vi "log analysis_gps.vi"() -> ()   [LabVIEW 2019] (continued)
11.7738,22.3000,0.0889,-0.2912,-0.0157,0.137018151,-1.334468427,280.534881050,0.4569,0.2986,0.5535,0.1156,0.0931,0.0772,0.0995,0.1050,4.8407,0f000001,0*4cc88e7a\n\tsystem status\tnormal 2 27.900000 0 0\trobot status\t339.401194\t32.171850\t11.773800\t0.137018\t-1.334468\t169.465119\t0.367000\t-0.094000\n\t\n15:29:25.3\tlog_raw\tgps_raw\t\tsystem status\tnormal 2 27.900000 0 0\trobot status\t339.281067\t32.209175\t11.771900\t0.263752\t-1.166349\t169.684950\t0.262000\t0.068000\n\t\n15:29:25.8\tlog_raw\tgps_raw\t#DUALANTENNAHEADINGA,USB3,0,50.0,FINESTEERING,2107,282583.800,02000000,d426,15824;SOL_COMPUTED,L1_FLOAT,-1.000000000,298.425811768,-39.243469238,0.0,360.000000000,180.000000000,\"631T\",12,4,4,4,04,00,20,00*99234be7\n\tsystem status\tnormal 2 27.900000 0 0\trobot status\t339.146863\t32.249468\t11.770100\t0.297724\t-0.965095\t169.902613\t0.288000\t0.022000\n\t\n15:29:26.3\tlog_raw\tgps_raw\t#INSPVAXA,USB3,0,50.0,FINESTEERING,2107,282584.350,02000000,471d,15824;INS_ALIGNMENT_COMPLETE,INS_RTKFIXED,37.37042121578,126.72466218098,11.7682,22.3000,0.0908,-0.2905,-0.0097,0.228953863,-0.969786949,279.904204523,0.4542,0.2977,0.5520,0.1156,0.0930,0.0771,0.0995,0.1050,4.8423,0f000001,0*25d05607\n\tsystem status\tnormal 2 27.900000 0 0\trobot status\t339.009591\t32.288365\t11.768300\t0.251734\t-1.037795\t170.066210\t0.264000\t0.046000\n\t\n15:29:26.8\tlog_raw\tgps_raw\t#DUALANTENNAHEADINGA,USB3,0,50.0,FINESTEERING,2107,282584.800,02000000,d426,15824;SOL_COMPUTED,L1_FLOAT,-1.000000000,317.813751221,-55.080688477,0.0,360.000000000,180.000000000,\"631T\",14,4,4,4,04,00,20,00*482add9e\n\tsystem status\tnormal 2 27.900000 0 0\trobot status\t338.871429\t32.326322\t11.766900\t0.026488\t-1.197862\t170.161249\t0.289000\t0.009000\n\t\n15:29:27.3\tlog_raw\tgps_raw\t#DUALANTENNAHEADINGA,USB3,0,47.5,FINESTEERING,2107,282585.300,02008000,d426,15824;SOL_COMPUTED,L1_FLOAT,-1.000000000,279.031005859,-12.437835693,0.0,360.000000000,180.000000000,\"631T\",14,4,4,4,04,00,20,00*e33ff00b\n\tsystem status\tnormal 2 28.000000 0 0\trobot status\t338.733347\t32.363284\t11.765300\t-0.055749\t-1.396296\t170.255636\t0.233000\t0.094000\n\t\n15:29:27.8\tlog_raw\tgps_raw\t#DUALANTENNAHEADINGA,USB3,0,47.5,FINESTEERING,2107,282585.800,02008000,d426,15824;SOL_COMPUTED,L1_FLOAT,-1.000000000,288.534484863,-28.210021973,0.0,360.000000000,180.000000000,\"631T\",14,4,4,4,04,00,20,00*75d90e5f\n\tsystem status\tnormal 2 28.000000 0 0\trobot status\t338.595043\t32.400275\t11.762200\t-0.027196\t-1.566060\t170.293366\t0.323000\t-0.045000\n\t\n15:29:28.3\tlog_raw\tgps_raw\t\tsystem status\tnormal 2 28.000000 0 0\trobot status\t338.457993\t32.437126\t11.760000\t0.076043\t-1.693350\t170.364624\t0.335000\t-0.046000\n\t\n15:29:28.8\tlog_raw\tgps_raw\t#DUALANTENNAHEADINGA,USB3,0,47.0,FINESTEERING,2107,282586.800,02008000,d426,15824;SOL_COMPUTED,L1_FLOAT,-1.000000000,299.638763428,-44.873535156,0.0,360.000000000,180.000000000,\"631T\",12,4,4,4,04,00,20,00*8433efc6\n\tsystem status\tnormal 2 28.000000 0 0\trobot status\t338.324624\t32.474153\t11.759800\t0.165974\t-1.454305\t170.318103\t0.343000\t-0.070000\n\t\n15:29:29.3\tlog_raw\tgps_raw\t\tsystem status\tnormal 2 28.000000 0 0\trobot status\t338.191330\t32.512553\t11.759700\t0.298969\t-1.287903\t170.233657\t0.318000\t-0.028000\n\t\n15:29:29.8\tlog_raw\tgps_raw\t#DUALANTENNAHEADINGA,USB3,0,51.0,FINESTEERING,2107,282587.800,02008000,d426,15824;SOL_COMPUTED,L1_FLOAT,-1.000000000,274.837402344,7.455324173,0.0,360.000000000,180.000000000,\"631T\",12,4,4,4,04,00,20,00*d357c890\n\tsystem status\tnormal 2 28.000000 0 0\trobot status\t338.054815\t32.551008\t11.758600\t0.166901\t-1.170996\t170.126054\t0.302000\t-0.007000\n\t\n15:29:30.3\tlog_raw\tgps_raw\t#INSPVAXA,USB3,0,53.0,FINESTEERING,2107,282588.350,02008000,471d,15824;INS_ALIGNMENT_COMPLETE,INS_RTKFIXED,37.37042392170,126.72464987629,11.7560,22.3000,0.0923,-0.2810,-0.0093,0.030566631,-0.932089530,279.991317390,0.4489,0.2966,0.5498,0.1150,0.0928,0.0771,0.0995,0.1049,4.8445,0f000001,0*cf0f29b3\n\tsystem status\tnormal 2 28.000000 0 0\trobot status\t337.906184\t32.592143\t11.756000\t0.030567\t-0.932090\t170.008683\t0.299000\t-0.010000\n\t\n15:29:30.8\tlog_raw\tgps_raw\t#DUALANTENNAHEADINGA,USB3,0,53.0,FINESTEERING,2107,282588.800,02008000,d426,15824;SOL_COMPUTED,L1_FLOAT,-1.000000000,322.314697266,-55.526092529,0.0,360.000000000,180.000000000,\"631T\",12,4,4,4,04,00,20,00*c23a8009\n\tsystem status\tnormal 2 28.000000 0 0\trobot status\t337.782114\t32.628114\t11.754100\t0.180332\t-1.046167\t169.865770\t0.297000\t-0.015000\n\t\n15:29:31.3\tlog_raw\tgps_raw\t#INSPVAXA,USB3,0,51.5,FINESTEERING,2107,282589.350,02000000,471d,15824;INS_ALIGNMENT_COMPLETE,INS_RTKFIXED,37.37042463832,126.72464679942,11.7536,22.3000,0.0961,-0.3116,-0.0160,0.320803902,-1.173970058,280.179307501,0.4487,0.2962,0.5495,0.1150,0.0928,0.0771,0.0995,0.1049,4.8450,0f000001,0*5f568f32\n\tsystem status\tnormal 2 28.000000 0 0\trobot status\t337.633639\t32.671688\t11.753600\t0.320804\t-1.173970\t169.820692\t0.309000\t-0.005000\n\t\n15:29:31.8\tlog_raw\tgps_raw\t#INSPVAXA,USB3,0,51.5,FINESTEERING,2107,282589.850,02000000,471d,15824;INS_ALIGNMENT_COMPLETE,INS_RTKFIXED,37.37042500999,126.72464523335,11.7530,22.3000,0.0866,-0.2870,-0.0118,0.410270840,-1.158910418,280.360984304,0.4487,0.2962,0.5495,0.1150,0.0928,0.0771,0.0995,0.1049,4.8450,0f000001,0*cae4522e\n\tsystem status\tnormal 2 28.000000 0 0\trobot status\t337.494920\t32.712944\t11.753000\t0.410271\t-1.158910\t169.639016\t0.295000\t-0.018000\n\t\n15:29:32.3\tlog_raw\tgps_raw\t#DUALANTENNAHEADINGA,USB3,0,50.5,FINESTEERING,2107,282590.300,02000000,d426,15824;INSUFFICIENT_OBS,NONE,-1.000000000,0.000000000,0.000000000,0.0,0.000000000,0.000000000,\"631T\",14,3,3,3,04,00,20,00*40a503c4\n\tsystem status\tnormal 2 28.000000 0 0\trobot status\t337.370086\t32.749840\t11.752800\t0.506298\t-1.276639\t169.454750\t0.298000\t-0.020000\n\t\n15:29:32.8\tlog_raw\tgps_raw\t\tsystem status\tnormal 2 28.000000 0 0\trobot status\t337.224367\t32.791209\t11.751600\t0.466373\t-1.308851\t169.314185\t0.301000\t-0.023000\n\t\n15:29:33.3\tlog_raw\tgps_raw\t#INSPVAXA,USB3,0,49.0,FINESTEERING,2107,282591.350,02000000,471d,15824;INS_ALIGNMENT_COMPLETE,INS_RTKFIXED,37.37042612746,126.72464043128,11.7509,22.3000,0.1112,-0.3046,-0.0107,0.438593312,-1.353837387,280.922848312,0.4465,0.2958,0.5485,0.1145,0.0928,0.0771,0.0995,0.1048,4.8451,0f000001,0*466c5cb5\n\tsystem status\tnormal 2 28.000000 0 0\trobot status\t337.069560\t32.836983\t11.750900\t0.438593\t-1.353837\t169.077152\t0.308000\t-0.006000\n\t\n15:29:33.8\tlog_raw\tgps_raw\t\tsystem status\tnormal 2 28.000000 0 0\trobot status\t336.938717\t32.876821\t11.750700\t0.385946\t-1.566220\t168.871041\t0.300000\t-0.020000\n\t\n15:29:34.3\tlog_raw\tgps_raw\t#INSPVAXA,USB3,0,48.0,FINESTEERING,2107,282592.350,02000000,471d,15824;INS_ALIGNMENT_COMPLETE,INS_RTKFIXED,37.37042693515,126.72463721970,11.7478,22.3000,0.1134,-0.2841,-0.0136,0.495116506,-1.748021922,281.445386324,0.4458,0.2955,0.5484,0.1143,0.0927,0.0771,0.0996,0.1048,4.8449,0f000001,0*7d422fc0\n\tsystem status\tnormal 2 28.000000 0 0\trobot status\t336.785084\t32.926635\t11.747800\t0.495117\t-1.748022\t168.554614\t0.242000\t-0.099000\n\t\n15:29:34.8\tlog_raw\tgps_raw\t\tsystem status\tnormal 2 28.000000 0 0\trobot status\t336.659133\t32.969106\t11.744800\t0.596199\t-1.886665\t168.112048\t0.349000\t0.047000\n\t\n15:29:35.3\tlog_raw\tgps_raw\t#INSPVAXA,USB3,0,51.5,FINESTEERING,2107,282593.350,02000000,471d,15824;INS_ALIGNMENT_COMPLETE,INS_RTKFIXED,37.37042777147,126.72463409939,11.7416,22.3000,0.1053,-0.2907,-0.0160,0.642644908,-1.933701573,282.530113202,0.4438,0.2953,0.5477,0.1141,0.0928,0.0771,0.0997,0.1048,4.8448,0f000001,0*602d795b\n\tsystem status\tnormal 2 27.900000 0 0\trobot status\t336.508692\t33.019465\t11.741600\t0.642645\t-1.933702\t167.469887\t0.298000\t-0.043000\n\t\n15:29:35.8\tlog_raw\tgps_raw\t#INSPVAXA,USB3,0,51.5,FINESTEERING,2107,282593.850,02000000,471d,15824;INS_ALIGNMENT_COMPLETE,INS_RTKFIXED,37.37042819780,126.72463255781,11.7390,22.3000,0.0952,-0.2916,-0.0106,0.650646949,-1.972506612,283.259305122,0.4438,0.2953,0.5477,0.1141,0.0928,0.0771,0.0997,0.1048,4.8448,0f000001,0*d7827024\n\tsystem status\tnormal 2 27.900000 0 0\trobot status\t336.372141\t33.066787\t11.739000\t0.650647\t-1.972507\t166.740695\t0.277000\t-0.054000\n\t\n15:29:36.3\tlog_raw\tgps_raw\t#INSPVAXA,USB3,0,49.5,FINESTEERING,2107,282594.350,02000000,471d,15824;INS_ALIGNMENT_COMPLETE,INS_RTKFIXED,37.37042864678,126.72463101246,11.7344,22.3000,0.0979,-0.2869,-0.0099,0.556878145,-1.878860029,284.055732763,0.4423,0.2949,0.5470,0.1139,0.0928,0.0770,0.0997,0.1048,4.8442,0f000001,0*f7248edf\n\tsystem status\tnormal 2 27.900000 0 0\trobot status\t336.235256\t33.116622\t11.734400\t0.556878\t-1.878860\t165.944267\t0.305000\t-0.016000\n\t\n15:29:36.8\tlog_raw\tgps_raw\t#INSPVAXA,USB3,0,49.5,FINESTEERING,2107,282594.850,02000000,471d,15824;INS_ALIGNMENT_COMPLETE,INS_RTKFIXED,37.37042912060,126.72462947652,11.7289,22.3000,0.1303,-0.2985,-0.0065,0.456318200,-1.931761270,284.972124281,0.4423,0.2949,0.5470,0.1139,0.0928,0.0770,0.0997,0.1048,4.8442,0f000001,0*61f64e67\n\tsystem status\tnormal 2 27.900000 0 0\trobot status\t336.099205\t33.169214\t11.728900\t0.456318\t-1.931761\t165.027876\t0.251000\t-0.124000\n\t\n15:29:37.3\tlog_raw\tgps_raw\t#INSPVAXA,USB3,0,48.5,FINESTEERING,2107,282595.350,02000000,471d,15824;INS_ALIGNMENT_COMPLETE,INS_RTKFIXED,37.37042961366,126.72462798098,11.7236,22.3000,0.1497,-0.2970,-0.0149,0.418327229,-1.868019582,285.752151928,0.4414,0.2947,0.5465,0.1139,0.0925,0.0770,0.0998,0.1049,4.8430,0f000001,0*1a617db7\n\tsystem status\tnormal 2 27.900000 0 0\trobot status\t335.966733\t33.223942\t11.723600\t0.418327\t-1.868020\t164.247848\t0.276000\t-0.063000\n\t\n15:29:37.8\tlog_raw\tgps_raw\t#INSPVAXA,USB3,0,48.5,FINESTEERING,2107,282595.850,02000000,471d,15824;INS_ALIGNMENT_COMPLETE,INS_RTKFIXED,37.37043014219,126.72462646518,11.7180,22.3000,0.1392,-0.2900,-0.0231,0.427669167,-1.922456438,286.476446001,0.4414,0.2947,0.5465,0.1139,0.0925,0.0770,0.0998,0.1049,4.8430,0f000001,0*1a66d065\n\tsystem status\tnormal 2 27.900000 0 0\trobot status\t335.832466\t33.282606\t11.718000\t0.427669\t-1.922456\t163.523554\t0.253000\t-0.085000\n\t\n15:29:38.3\tlog_raw\tgps_raw\t#INSPVAXA,USB3,0,50.5,FINESTEERING,2107,282596.350,02000000,471d,15824;INS_ALIGNMENT_COMPLETE,INS_RTKFIXED,37.37043069447,126.72462494509,11.7122,22.3000,0.1569,-0.2925,-0.0148,0.456002187,-2.188056466,287.205419298,0.4412,0.2946,0.5461,0.1139,0.0925,0.0770,0.0999,0.1050,4.8425,0f000001,0*15a09225\n\tsystem status\tnormal 2 27.900000 0 0\trobot status\t335.697819\t33.343906\t11.712200\t0.456002\t-2.188056\t162.794581\t0.332000\t0.022000\n\t\n15:29:38.8\tlog_raw\tgps_raw\t#INSPVAXA,USB3,0,50.5,FINESTEERING,2107,282596.850,02000000,471d,15824;INS_ALIGNMENT_COMPLETE,INS_RTKFIXED,37.37043125589,126.72462344785,11.7060,22.3000,0.1402,-0.2734,-0.0172,0.395468070,-2.411480135,287.743907623,0.4412,0.2946,0.5461,0.1139,0.0925,0.0770,0.0999,0.1050,4.8425,0f000001,0*9ae986ea\n\tsystem status\tnormal 2 27.900000 0 0\trobot status\t335.565196\t33.406220\t11.706000\t0.395468\t-2.411480\t162.256092\t0.351000\t0.058000\n\t\n15:29:39.3\tlog_raw\tgps_raw\t#INSPVAXA,USB3,0,49.0,FINESTEERING,2107,282597.350,02000000,471d,15824;INS_ALIGNMENT_COMPLETE,INS_RTKFIXED,37.37043180809,126.72462197460,11.7004,22.3000,0.1451,-0.2798,-0.0240,0.082189404,-2.342857619,288.211463548,0.4406,0.2943,0.5456,0.1138,0.0925,0.0770,0.1000,0.1050,4.8425,0f000001,0*a4baef99\n\tsystem status\tnormal 2 27.900000 0 0\trobot status\t335.434698\t33.467511\t11.700400\t0.082189\t-2.342858\t161.788536\t0.329000\t0.043000\n\t\n15:29:39.8\tlog_raw\tgps_raw\t\tsystem status\tnormal 2 27.900000 0 0\trobot status\t335.317862\t33.526109\t11.695100\t0.085459\t-2.333479\t161.447051\t0.248000\t-0.071000\n\t\n15:29:40.3\tlog_raw\tgps_raw\t#INSPVAXA,USB3,0,47.0,FINESTEERING,2107,282598.350,02000000,471d,15824;INS_ALIGNMENT_COMPLETE,INS_RTKFIXED,37.37043296335,126.72461906573,11.6872,22.3000,0.1639,-0.2709,-0.0144,0.075715172,-2.060890876,288.886128801,0.4401,0.2937,0.5452,0.1138,0.0925,0.0770,0.1001,0.1051,4.8435,0f000001,0*53c08aab\n\tsystem status\tnormal 2 28.000000 0 0\trobot status\t335.177035\t33.595737\t11.687200\t0.075715\t-2.060891\t161.113871\t0.246000\t-0.079000\n\t\n15:29:40.8\tlog_raw\tgps_raw\t#INSPVAXA,USB3,0,47.0,FINESTEERING,2107,282598.850,02000000,471d,15824;INS_ALIGNMENT_COMPLETE,INS_RTKFIXED,37.37043354014,126.72461760390,11.6788,22.3000,0.1599,-0.2669,-0.0128,0.049311349,-2.026534390,289.114340802,0.4401,0.2937,0.5452,0.1138,0.0925,0.0770,0.1001,0.1051,4.8435,0f000001,0*6b176d5a\n\tsystem status\tnormal 2 28.000000 0 0\trobot status\t335.047548\t33.659757\t11.678800\t0.049311\t-2.026534\t160.885659\t0.254000\t-0.066000\n\t\n15:29:41.3\tlog_raw\tgps_raw\t#INSPVAXA,USB3,0,48.5,FINESTEERING,2107,282599.350,02000000,471d,15824;INS_ALIGNMENT_COMPLETE,INS_RTKFIXED,37.37043410493,126.72461616545,11.6719,22.3000,0.1624,-0.2885,-0.0138,-0.156644949,-2.114929380,289.341942256,0.4397,0.2935,0.5448,0.1139,0.0926,0.0770,0.1001,0.1052,4.8449,0f000001,0*992413bc\n\tsystem status\tnormal 2 28.000000 0 0\trobot status\t334.920133\t33.722445\t11.671900\t-0.156645\t-2.114929\t160.658058\t0.305000\t0.006000\n\t\n15:29:41.8\tlog_raw\tgps_raw\t#INSPVAXA,USB3,0,48.5,FINESTEERING,2107,282599.850,02000000,471d,15824;INS_ALIGNMENT_COMPLETE,INS_RTKFIXED,37.37043467790,126.72461472498,11.6664,22.3000,0.1607,-0.2703,-0.0125,-0.362948004,-2.133534264,289.548423016,0.4397,0.2935,0.5448,0.1139,0.0926,0.0770,0.1001,0.1052,4.8449,0f000001,0*c10a254e\n\tsystem status\tnormal 2 28.000000 0 0\trobot status\t334.792538\t33.786041\t11.666400\t-0.362948\t-2.133534\t160.451577\t0.297000\t0.000000\n\t\n15:29:42.3\tlog_raw\tgps_raw\t#INSPVAXA,USB3,0,49.5,FINESTEERING,2107,282600.350,02000000,471d,15824;INS_ALIGNMENT_COMPLETE,INS_RTKFIXED,37.37043525953,126.72461325909,11.6615,22.3000,0.1615,-0.2803,-0.0148,-0.471431775,-2.267846962,289.732073791,0.4392,0.2934,0.5443,0.1138,0.0928,0.0769,0.1001,0.1052,4.8460,0f000001,0*36a380c0\n\tsystem status\tnormal 2 28.000000 0 0\trobot status\t334.662692\t33.850598\t11.661500\t-0.471432\t-2.267847\t160.267926\t0.302000\t0.012000\n\t\n15:29:42.8\tlog_raw\tgps_raw\t#INSPVAXA,USB3,0,49.5,FINESTEERING,2107,282600.850,02000000,471d,15824;INS_ALIGNMENT_COMPLETE,INS_RTKFIXED,37.37043586783,126.72461175288,11.6568,22.3000,0.1684,-0.2866,-0.0132,-0.451303759,-2.269558677,289.856432048,0.4392,0.2934,0.5443,0.1138,0.0928,0.0769,0.1001,0.1052,4.8460,0f000001,0*3d745bd7\n\tsystem status\tnormal 2 28.000000 0 0\trobot status\t334.529274\t33.918116\t11.656800\t-0.451304\t-2.269559\t160.143568\t0.307000\t0.003000\n\t\n15:29:43.3\tlog_raw\tgps_raw\t#INSPVAXA,USB3,0,47.5,FINESTEERING,2107,282601.350,02000000,471d,15824;INS_ALIGNMENT_COMPLETE,INS_RTKFIXED,37.37043647524,126.72461026809,11.6515,22.3000,0.1700,-0.2809,-0.0124,-0.328241253,-2.248777073,289.979230408,0.4390,0.2932,0.5439,0.1138,0.0927,0.0769,0.1000,0.1052,4.8467,0f000001,0*88c87769\n\tsystem status\tnormal 2 28.000000 0 0\trobot status\t334.397754\t33.985534\t11.651500\t-0.328241\t-2.248777\t160.020770\t0.296000\t0.009000\n\t\n15:29:43.8\tlog_raw\tgps_raw\t#INSPVAXA,USB3,0,47.5,FINESTEERING,2107,282601.850,02000000,471d,15824;INS_ALIGNMENT_COMPLETE,INS_RTKFIXED,37.37043706474,126.72460883352,11.6472,22.3000,0.1674,-0.2631,-0.0107,-0.295120633,-2.255482926,290.118733293,0.4390,0.2932,0.5439,0.1138,0.0927,0.0769,0.1000,0.1052,4.8467,0f000001,0*60fbd16c\n\tsystem status\tnormal 2 28.000000 0 0\trobot status\t334.270682\t34.050965\t11.647200\t-0.295121\t-2.255483\t159.881267\t0.294000\t0.009000\n\t\n15:29:44.3\tlog_raw\tgps_raw\t#INSPVAXA,USB3,0,49.5,FINESTEERING,2107,282602.350,02000000,471d,15824;INS_ALIGNMENT_COMPLETE,INS_RTKFIXED,37.37043766543,126.72460736241,11.6426,22.3000,0.1773,-0.2821,-0.0125,-0.322654423,-2.363199962,290.226882800,0.4388,0.2931,0.5437,0.1138,0.0926,0.0769,0.0999,0.1052,4.8468,0f000001,0*f3791758\n\tsystem status\tnormal 2 28.000000 0 0\trobot status\t334.140374\t34.117637\t11.642600\t-0.322654\t-2.363200\t159.773117\t0.298000\t0.000000\n\t\n15:29:44.8\tlog_raw\tgps_raw\t#INSPVAXA,USB3,0,49.5,FINESTEERING,2107,282602.850,02000000,471d,15824;INS_ALIGNMENT_COMPLETE,INS_RTKFIXED,37.37043827005,126.72460590169,11.6385,22.3000,0.1821,-0.2724,-0.0121,-0.418675445,-2.261623622,290.351055865,0.4388,0.2931,0.5437,0.1138,0.0926,0.0769,0.0999,0.1052,4.8468,0f000001,0*204debac\n\tsystem status\tnormal 2 28.000000 0 0\trobot status\t334.010986\t34.184746\t11.638500\t-0.418675\t-2.261624\t159.648944\t0.294000\t-0.001000\n\t\n15:29:45.3\tlog_raw\tgps_raw\t#INSPVAXA,USB3,0,44.5,FINESTEERING,2107,282603.350,02000000,471d,15824;INS_ALIGNMENT_COMPLETE,INS_RTKFIXED,37.37043885036,126.72460451664,11.6355,22.3000,0.1725,-0.2572,-0.0117,-0.454843723,-2.160794151,290.461374575,0.4389,0.2930,0.5435,0.1139,0.0927,0.0769,0.0999,0.1052,4.8469,0f000001,0*fe35c8bb\n\tsystem status\tnormal 2 28.000000 0 0\trobot status\t333.888300\t34.249156\t11.635500\t-0.454844\t-2.160794\t159.538625\t0.291000\t0.005000\n\t\n15:29:45.8\tlog_raw\tgps_raw\t#INSPVAXA,USB3,0,44.5,FINESTEERING,2107,282603.850,02000000,471d,15824;INS_ALIGNMENT_COMPLETE,INS_RTKFIXED,37.37043945299,126.72460307083,11.6317,22.3000,0.1803,-0.2729,-0.0125,-0.455229843,-2.077941582,290.572474787,0.4389,0.2930,0.5435,0.1139,0.0927,0.0769,0.0999,0.1052,4.8469,0f000001,0*cc614426\n\tsystem status\tnormal 2 28.000000 0 0\trobot status\t333.760233\t34.316044\t11.631700\t-0.455230\t-2.077942\t159.427525\t0.296000\t-0.001000\n\t\n15:29:46.3\tlog_raw\tgps_raw\t#INSPVAXA,USB3,0,48.5,FINESTEERING,2107,282604.350,02000000,471d,15824;INS_ALIGNMENT_COMPLETE,INS_RTKFIXED,37.37044007383,126.72460154659,11.6273,22.3000,0.1929,-0.2951,-0.0109,-0.392288663,-2.045966583,290.664646635,0.4392,0.2930,0.5434,0.1140,0.0926,0.0769,0.0998,0.1052,4.8464,0f000001,0*8e2e8e57\n\tsystem status\tnormal 2 28.000000 0 0\trobot status\t333.625218\t34.384953\t11.627300\t-0.392289\t-2.045967\t159.335353\t0.305000\t-0.014000\n\t\n15:29:46.8\tlog_raw\tgps_raw\t\tsystem status\tnormal 2 28.000000 0 0\trobot status\t333.495549\t34.451599\t11.623100\t-0.365595\t-2.059636\t159.140144\t0.289000\t-0.003000\n\t\n15:29:47.3\tlog_raw\tgps_raw\t\tsystem status\tnormal 2 28.000000 0 0\trobot status\t333.374797\t34.512807\t11.619700\t-0.496135\t-2.084050\t159.003990\t0.295000\t-0.006000\n\t\n15:29:47.8\tlog_raw\tgps_raw\t#INSPVAXA,USB3,0,46.0,FINESTEERING,2107,282605.850,02000000,471d,15824;INS_ALIGNMENT_COMPLETE,INS_RTKFIXED,37.37044182670,126.72459720127,11.6153,22.3000,0.1906,-0.2962,-0.0097,-0.601316831,-2.333994849,291.196527762,0.4394,0.2930,0.5433,0.1141,0.0926,0.0769,0.0997,0.1052,4.8458,0f000001,0*9a6d08c1\n\tsystem status\tnormal 2 28.000000 0 0\trobot status\t333.240317\t34.579510\t11.615300\t-0.601317\t-2.333995\t158.803472\t0.310000\t-0.005000\n\t\n15:29:48.3\tlog_raw\tgps_raw\t#INSPVAXA,USB3,0,47.0,FINESTEERING,2107,282606.350,02000000,471d,15824;INS_ALIGNMENT_COMPLETE,INS_RTKFIXED,37.37044241168,126.72459579253,11.6120,22.3000,0.1650,-0.2486,-0.0027,-0.608391314,-2.324818349,291.383905054,0.4412,0.2932,0.5437,0.1140,0.0926,0.0769,0.0996,0.1052,4.8446,0f000001,0*3d88472b\n\tsystem status\tnormal 2 28.000000 0 0\trobot status\t333.115533\t34.644439\t11.612000\t-0.608391\t-2.324818\t158.616095\t0.296000\t-0.024000\n\t\n15:29:48.8\tlog_raw\tgps_raw\t#INSPVAXA,USB3,0,47.0,FINESTEERING,2107,282606.850,02000000,471d,15824;INS_ALIGNMENT_COMPLETE,INS_RTKFIXED,37.37044299863,126.72459438872,11.6086,22.3000,0.1967,-0.2948,-0.0098,-0.716784784,-2.185835585,291.603581988,0.4412,0.2932,0.5437,0.1140,0.0926,0.0769,0.0996,0.1052,4.8446,0f000001,0*5390b691\n\tsystem status\tnormal 2 28.000000 0 0\trobot status\t332.991186\t34.709586\t11.608600\t-0.716785\t-2.185836\t158.396418\t0.323000\t0.004000\n\t\n15:29:49.3\tlog_raw\tgps_raw\t#INSPVAXA,USB3,0,50.5,FINESTEERING,2107,282607.350,02000000,471d,15824;INS_ALIGNMENT_COMPLETE,INS_RTKFIXED,37.37044361320,126.72459293136,11.6060,22.3000,0.1791,-0.2405,0.0044,-0.624652897,-2.258872249,291.867019396,0.4427,0.2934,0.5443,0.1141,0.0925,0.0769,0.0996,0.1052,4.8437,0f000001,0*4de0af31\n\tsystem status\tnormal 2 28.000000 0 0\trobot status\t332.862095\t34.777799\t11.606000\t-0.624653\t-2.258872\t158.132981\t0.249000\t-0.072000\n\t\n15:29:49.8\tlog_raw\tgps_raw\t#INSPVAXA,USB3,0,50.5,FINESTEERING,2107,282607.850,02000000,471d,15824;INS_ALIGNMENT_COMPLETE,INS_RTKFIXED,37.37044423988,126.72459145739,11.6024,22.3000,0.1844,-0.2484,-0.0073,-0.519908618,-2.368148317,292.226693813,0.4427,0.2934,0.5443,0.1141,0.0925,0.0769,0.0996,0.1052,4.8437,0f000001,0*603a82db\n\tsystem status\tnormal 2 28.000000 0 0\trobot status\t332.731533\t34.847356\t11.602400\t-0.519909\t-2.368148\t157.773306\t0.280000\t-0.046000\n\t\n15:29:50.3\tlog_raw\tgps_raw\t#INSPVAXA,USB3,0,51.0,FINESTEERING,2107,282608.350,02000000,471d,15824;INS_ALIGNMENT_COMPLETE,INS_RTKFIXED,37.37044483752,126.72459005434,11.5979,22.3000,0.1715,-0.2554,-0.0122,-0.519117149,-2.380892114,292.717494679,0.4421,0.2933,0.5443,0.1142,0.0925,0.0769,0.0995,0.1051,4.8434,0f000001,0*764df120\n\tsystem status\tnormal 2 28.000000 0 0\trobot status\t332.607253\t34.913690\t11.597900\t-0.519117\t-2.380892\t157.282505\t0.259000\t-0.079000\n\t\n15:29:50.8\tlog_raw\tgps_raw\t\tsystem status\tnormal 2 27.900000 0 0\trobot status\t332.481353\t34.981067\t11.593400\t-0.588090\t-2.482163\t156.720993\t0.356000\t0.045000\n\t\n15:29:51.3\tlog_raw\tgps_raw\t#INSPVAXA,USB3,0,47.0,FINESTEERING,2107,282609.350,02000000,471d,15824;INS_ALIGNMENT_COMPLETE,INS_RTKFIXED,37.37044605652,126.72458722854,11.5885,22.3000,0.1663,-0.2764,-0.0069,-0.648305418,-2.537713416,293.939898101,0.4422,0.2933,0.5445,0.1140,0.0925,0.0769,0.0995,0.1051,4.8432,0f000001,0*830d3839\n\tsystem status\tnormal 2 27.900000 0 0\trobot status\t332.356949\t35.048990\t11.588500\t-0.648305\t-2.537713\t156.060102\t0.252000\t-0.093000\n\t\n15:29:51.8\tlog_raw\tgps_raw\t\tsystem status\tnormal 2 27.900000 0 0\trobot status\t332.232042\t35.119047\t11.582700\t-0.745254\t-2.693669\t155.334559\t0.251000\t-0.106000\n\t\n15:29:52.3\tlog_raw\tgps_raw\t#INSPVAXA,USB3,0,49.0,FINESTEERING,2107,282610.350,02000000,471d,15824;INS_ALIGNMENT_COMPLETE,INS_RTKFIXED,37.37044732236,126.72458446831,11.5778,22.3000,0.1884,-0.2557,-0.0029,-0.876321406,-2.449391486,295.430567939,0.4418,0.2933,0.5445,0.1139,0.0924,0.0769,0.0995,0.1051,4.8434,0f000001,0*8a5ecd23\n\tsystem status\tnormal 2 27.900000 0 0\trobot status\t332.112452\t35.189488\t11.577800\t-0.876321\t-2.449391\t154.569432\t0.313000\t-0.017000\n\t\n15:29:52.8\tlog_raw\tgps_raw\t\tsystem status\tnormal 2 27.900000 0 0\trobot status\t331.995619\t35.262702\t11.573300\t-0.747535\t-2.269714\t153.755206\t0.285000\t-0.046000\n\t\n15:29:53.3\tlog_raw\tgps_raw\t#INSPVAXA,USB3,0,48.5,FINESTEERING,2107,282611.350,02000000,471d,15824;INS_ALIGNMENT_COMPLETE,INS_RTKFIXED,37.37044865428,126.72458179844,11.5688,22.3000,0.1893,-0.2465,-0.0147,-0.836892789,-2.139837911,297.111108164,0.4413,0.2932,0.5444,0.1139,0.0924,0.0769,0.0995,0.1050,4.8437,0f000001,0*5c5081ba\n\tsystem status\tnormal 2 27.900000 0 0\trobot status\t331.875959\t35.337320\t11.568800\t-0.836893\t-2.139838\t152.888892\t0.350000\t0.052000\n\t\n15:29:53.8\tlog_raw\tgps_raw\t\tsystem status\tnormal 2 27.900000 0 0\trobot status\t331.759057\t35.412285\t11.564500\t-0.960199\t-1.953891\t152.039743\t0.246000\t-0.102000\n\t\n15:29:54.3\tlog_raw\tgps_raw\t#INSPVAXA,USB3,0,49.0,FINESTEERING,2107,282612.350,02000000,471d,15824;INS_ALIGNMENT_COMPLETE,INS_RTKFIXED,37.37045003475,126.72457914119,11.5590,22.3000,0.1912,-0.2423,-0.0135,-1.077738591,-1.947492637,298.710847895,0.4411,0.2932,0.5444,0.1142,0.0925,0.0769,0.0995,0.1050,4.8438,0f000001,0*1786ad92\n\tsystem status\tnormal 2 27.900000 0 0\trobot status\t331.640584\t35.490541\t11.559000\t-1.077739\t-1.947493\t151.289152\t0.302000\t0.002000\n\t\n15:29:54.8\tlog_raw\tgps_raw\t\tsystem status\tnormal 2 27.900000 0 0\trobot status\t331.519484\t35.572483\t11.553300\t-1.146376\t-2.235984\t150.679646\t0.277000\t-0.033000\n\t\n15:29:55.3\tlog_raw\tgps_raw\t#INSPVAXA,USB3,0,51.5,FINESTEERING,2107,282613.350,02000000,471d,15824;INS_ALIGNMENT_COMPLETE,INS_RTKFIXED,37.37045149851,126.72457646585,11.5487,22.3000,0.1950,-0.2536,-0.0123,-1.258648342,-2.137744772,299.825187137,0.4411,0.2932,0.5443,0.1140,0.0925,0.0769,0.0994,0.1050,4.8434,0f000001,0*52f4ee79\n\tsystem status\tnormal 2 27.900000 0 0\trobot status\t331.403607\t35.653005\t11.548700\t-1.258648\t-2.137745\t150.174813\t0.234000\t-0.119000\n\t\n15:29:55.8\tlog_raw\tgps_raw\t\tsystem status\tnormal 2 28.000000 0 0\trobot status\t331.288824\t35.735706\t11.544600\t-1.273791\t-2.256592\t149.724950\t0.366000\t0.087000\n\t\n15:29:56.3\tlog_raw\tgps_raw\t#INSPVAXA,USB3,0,46.0,FINESTEERING,2107,282614.350,02000000,471d,15824;INS_ALIGNMENT_COMPLETE,INS_RTKFIXED,37.37045301719,126.72457385904,11.5391,22.3000,0.2078,-0.2477,-0.0088,-1.293609252,-2.271198924,300.637369153,0.4405,0.2931,0.5441,0.1140,0.0925,0.0769,0.0994,0.1049,4.8428,0f000001,0*b4115fbd\n\tsystem status\tnormal 2 27.900000 0 0\trobot status\t331.172700\t35.821564\t11.539100\t-1.293609\t-2.271199\t149.362631\t0.313000\t0.005000\n\t\n15:29:56.8\tlog_raw\tgps_raw\t\tsystem status\tnormal 2 28.000000 0 0\trobot status\t331.060259\t35.906870\t11.532800\t-1.322364\t-1.872346\t149.068529\t0.251000\t-0.066000\n\t\n15:29:57.3\tlog_raw\tgps_raw\t#INSPVAXA,USB3,0,50.0,FINESTEERING,2107,282615.350,02000000,471d,15824;INS_ALIGNMENT_COMPLETE,INS_RTKFIXED,37.37045455007,126.72457134249,11.5267,22.3000,0.2142,-0.2258,-0.0244,-1.294164682,-1.774661927,301.229016667,0.4401,0.2931,0.5440,0.1144,0.0926,0.0769,0.0994,0.1049,4.8422,0f000001,0*3cd07d07\n\tsystem status\tnormal 2 28.000000 0 0\trobot status\t330.949788\t35.991699\t11.526700\t-1.294165\t-1.774662\t148.770983\t0.399000\t0.147000\n\t\n15:29:57.8\tlog_raw\tgps_raw\t\tsystem status\tnormal 2 28.000000 0 0\trobot status\t330.837032\t36.078184\t11.520900\t-1.287493\t-1.883163\t148.532510\t0.241000\t-0.076000\n\t\n15:29:58.3\tlog_raw\tgps_raw\t\tsystem status\tnormal 2 28.000000 0 0\trobot status\t330.722226\t36.167303\t11.515200\t-1.217293\t-1.953965\t148.289410\t0.353000\t0.076000\n\t\n15:29:58.8\tlog_raw\tgps_raw\t\tsystem status\tnormal 2 28.000000 0 0\trobot status\t330.609570\t36.256371\t11.509900\t-1.198936\t-2.148076\t148.089006\t0.292000\t-0.010000\n\t\n15:29:59.3\tlog_raw\tgps_raw\t\tsystem status\tnormal 2 28.000000 0 0\trobot status\t330.495889\t36.345741\t11.504200\t-1.214097\t-2.229590\t147.895949\t0.294000\t-0.006000\n\t\n15:29:59.8\tlog_raw\tgps_raw\t\tsystem status\tnormal 2 28.000000 0 0\trobot status\t330.384976\t36.433703\t11.498200\t-1.195726\t-2.093029\t147.680567\t0.304000\t0.007000\n\t\n15:30:00.3\tlog_raw\tgps_raw\t\tsystem status\tnormal 2 28.000000 0 0\trobot status\t330.267550\t36.525284\t11.491200\t-1.171973\t-2.202935\t147.472403\t0.303000\t0.000000\n\t\n15:30:00.8\tlog_raw\tgps_raw\t\tsystem status\tnormal 2 28.000000 0 0\trobot status\t330.153094\t36.615290\t11.483800\t-1.107828\t-2.295701\t147.276575\t0.275000\t-0.033000\n\t\n15:30:01.3\tlog_raw\tgps_raw\t\tsystem status\tnormal 2 28.000000 0 0\trobot status\t330.048177\t36.698148\t11.477700\t-1.024468\t-2.175771\t147.115099\t0.289000\t-0.003000\n\t\n15:30:01.8\tlog_raw\tgps_raw\t\tsystem status\tnormal 2 28.000000 0 0\trobot status\t329.932232\t36.786766\t11.472000\t-1.033546\t-2.355252\t146.955217\t0.302000\t0.004000\n\t\n15:30:02.3\tlog_raw\tgps_raw\t#INSPVAXA,USB3,0,50.5,FINESTEERING,2107,282620.350,02000000,471d,15824;INS_ALIGNMENT_COMPLETE,INS_RTKFIXED,37.37046253392,126.72455852077,11.4659,22.3000,0.2027,-0.2268,-0.0270,-1.031833865,-2.375437300,303.226270712,0.4405,0.2931,0.5444,0.1138,0.0928,0.0769,0.0992,0.1046,4.8369,0f000001,0*42a616f1\n\tsystem status\tnormal 2 28.000000 0 0\trobot status\t329.814061\t36.877828\t11.465900\t-1.031834\t-2.375437\t146.773729\t0.295000\t-0.002000\n\t\n15:30:02.8\tlog_raw\tgps_raw\t\tsystem status\tnormal 2 28.000000 0 0\trobot status\t329.701199\t36.966164\t11.459100\t-1.012014\t-2.169479\t146.633342\t0.302000\t0.001000\n\t\n15:30:03.3\tlog_raw\tgps_raw\t\tsystem status\tnormal 2 28.000000 0 0\trobot status\t329.587202\t37.055061\t11.451900\t-0.984894\t-2.154782\t146.517827\t0.285000\t0.024000\n\t\n15:30:03.8\tlog_raw\tgps_raw\t\tsystem status\tnormal 2 28.000000 0 0\trobot status\t329.473134\t37.142553\t11.445200\t-1.073548\t-2.160210\t146.375568\t0.298000\t0.004000\n\t\n15:30:04.3\tlog_raw\tgps_raw\t\tsystem status\tnormal 2 28.000000 0 0\trobot status\t329.359768\t37.229625\t11.439600\t-1.167303\t-2.070061\t146.268267\t0.292000\t0.012000\n\t\n15:30:04.8\tlog_raw\tgps_raw\t\tsystem status\tnormal 2 28.000000 0 0\trobot status\t329.249168\t37.315142\t11.435000\t-1.146874\t-2.103983\t146.153177\t0.296000\t0.006000\n\t\n15:30:05.3\tlog_raw\tgps_raw\t\tsystem status\tnormal 2 28.000000 0 0\trobot status\t329.141006\t37.398576\t11.429900\t-1.193837\t-2.089631\t146.016308\t0.301000\t0.000000\n\t\n15:30:05.8\tlog_raw\tgps_raw\t#INSPVAXA,USB3,0,49.5,FINESTEERING,2107,282623.850,02000000,471d,15824;INS_ALIGNMENT_COMPLETE,INS_RTKFIXED,37.37046800824,126.72454964821,11.4249,22.3000,0.1899,-0.2361,-0.0160,-1.285475051,-1.943866845,304.127219371,0.4404,0.2931,0.5447,0.1139,0.0925,0.0769,0.0992,0.1044,4.8359,0f000001,0*b0ab9613\n\tsystem status\tnormal 2 28.000000 0 0\trobot status\t329.028144\t37.485424\t11.424900\t-1.285475\t-1.943867\t145.872781\t0.298000\t-0.002000\n\t\n15:30:06.3\tlog_raw\tgps_raw\t\tsystem status\tnormal 2 28.000000 0 0\trobot status\t328.915105\t37.574636\t11.420900\t-1.317138\t-1.904264\t145.782482\t0.302000\t0.000000\n\t\n15:30:06.8\tlog_raw\tgps_raw\t\tsystem status\tnormal 2 28.000000 0 0\trobot status\t328.802525\t37.664668\t11.417300\t-1.308606\t-1.947832\t145.748217\t0.249000\t0.074000\n\t\n15:30:07.3\tlog_raw\tgps_raw\t\tsystem status\tnormal 2 28.000000 0 0\trobot status\t328.689331\t37.755365\t11.414500\t-1.335730\t-1.912686\t145.714457\t0.284000\t0.024000\n\t\n15:30:07.8\tlog_raw\tgps_raw\t\tsystem status\tnormal 2 28.000000 0 0\trobot status\t328.579616\t37.844346\t11.412900\t-1.260212\t-1.843256\t145.734421\t0.251000\t0.066000\n\t\n15:30:08.3\tlog_raw\tgps_raw\t\tsystem status\tnormal 2 28.000000 0 0\trobot status\t328.468951\t37.933977\t11.410900\t-1.181111\t-1.711309\t145.781602\t0.263000\t0.059000\n\t\n15:30:08.8\tlog_raw\tgps_raw\t\tsystem status\tnormal 2 28.000000 0 0\trobot status\t328.357086\t38.023949\t11.408300\t-1.193237\t-1.626801\t145.892575\t0.314000\t-0.009000\n\t\n15:30:09.3\tlog_raw\tgps_raw\t\tsystem status\tnormal 2 28.000000 0 0\trobot status\t328.243998\t38.114237\t11.405400\t-1.246737\t-1.595534\t146.062386\t0.300000\t-0.003000\n\t\n15:30:09.8\tlog_raw\tgps_raw\t\tsystem status\tnormal 2 28.000000 0 0\trobot status\t328.132302\t38.204673\t11.403200\t-1.147078\t-1.598318\t146.223974\t0.309000\t-0.009000\n\t\n15:30:10.3\tlog_raw\tgps_raw\t\tsystem status\tnormal 2 27.900000 0 0\trobot status\t328.021416\t38.294788\t11.401400\t-1.008413\t-1.706250\t146.381148\t0.255000\t0.080000\n\t\n15:30:10.8\tlog_raw\tgps_raw\t\tsystem status\tnormal 2 28.000000 0 0\trobot status\t327.906592\t38.385568\t11.398800\t-1.115508\t-1.910397\t146.512211\t0.419000\t-0.160000\n\t\n15:30:11.3\tlog_raw\tgps_raw\t\tsystem status\tnormal 2 28.000000 0 0\trobot status\t327.794397\t38.476197\t11.394500\t-1.066882\t-2.089226\t146.594877\t0.244000\t0.092000\n\t\n15:30:11.8\tlog_raw\tgps_raw\t\tsystem status\tnormal 2 27.900000 0 0\trobot status\t327.684237\t38.565339\t11.390100\t-1.090959\t-2.090633\t146.729691\t0.250000\t0.066000\n\t\n15:30:12.3\tlog_raw\tgps_raw\t\tsystem status\tnormal 2 28.000000 0 0\trobot status\t327.573329\t38.656076\t11.387900\t-1.054905\t-2.062997\t146.864014\t0.304000\t-0.013000\n\t\n15:30:12.9\tlog_raw\tgps_raw\t\tsystem status\tnormal 2 28.000000 0 0\trobot status\t327.460090\t38.748598\t11.385800\t-1.065738\t-2.203317\t146.996303\t0.474000\t-0.264000\n\t\n15:30:13.4\tlog_raw\tgps_raw\t\tsystem status\tnormal 2 28.000000 0 0\trobot status\t327.350714\t38.837872\t11.383500\t-1.077778\t-2.097281\t147.088314\t0.336000\t-0.062000\n\t\n15:30:13.9\tlog_raw\tgps_raw\t\tsystem status\tnormal 2 28.000000 0 0\trobot status\t327.240362\t38.927323\t11.381300\t-1.132156\t-2.039123\t147.271649\t0.370000\t-0.096000\n\t\n15:30:14.4\tlog_raw\tgps_raw\t\tsystem status\tnormal 2 28.000000 0 0\trobot status\t327.128264\t39.017718\t11.378200\t-1.133717\t-2.133654\t147.344781\t0.280000\t0.036000\n\t\n15:30:14.9\tlog_raw\tgps_raw\t\tsystem status\tnormal 2 28.000000 0 0\trobot status\t327.016896\t39.108573\t11.375700\t-1.043724\t-2.163807\t147.485179\t0.398000\t-0.129000\n\t\n15:30:15.4\tlog_raw\tgps_raw\t\tsystem status\tnormal 2 28.000000 0 0\trobot status\t326.907685\t39.197108\t11.373400\t-1.100464\t-2.036859\t147.609527\t0.262000\t0.071000\n\t\n15:30:15.9\tlog_raw\tgps_raw\t\tsystem status\tnormal 2 28.000000 0 0\trobot status\t326.794587\t39.287565\t11.371200\t-1.261829\t-2.138646\t147.755480\t0.278000\t0.045000\n\t\n15:30:16.4\tlog_raw\tgps_raw\t\tsystem status\tnormal 2 28.000000 0 0\trobot status\t326.682213\t39.377127\t11.369800\t-1.311056\t-1.954493\t147.886689\t0.243000\t0.092000\n\t\n15:30:16.9\tlog_raw\tgps_raw\t\tsystem status\tnormal 2 28.000000 0 0\trobot status\t326.570964\t39.465579\t11.368500\t-1.310622\t-1.814417\t148.011818\t0.283000\t0.034000\n\t\n15:30:17.4\tlog_raw\tgps_raw\t\tsystem status\tnormal 2 28.000000 0 0\trobot status\t326.458417\t39.552955\t11.366300\t-1.427487\t-1.811345\t148.176140\t0.231000\t0.119000\n\t\n15:30:17.9\tlog_raw\tgps_raw\t\tsystem status\tnormal 2 27.900000 0 0\trobot status\t326.344998\t39.641504\t11.363300\t-1.401160\t-1.801691\t148.293640\t0.451000\t-0.219000\n\t\n15:30:18.4\tlog_raw\tgps_raw\t\tsystem status\tnormal 2 28.000000 0 0\trobot status\t326.230871\t39.728945\t11.360100\t-1.542371\t-1.881234\t148.394701\t0.237000\t0.094000\n\t\n15:30:18.9\tlog_raw\tgps_raw\t\tsystem status\tnormal 2 27.900000 0 0\trobot status\t326.118208\t39.816512\t11.356700\t-1.546773\t-2.081995\t148.503000\t0.216000\t0.130000\n\t\n15:30:19.4\tlog_raw\tgps_raw\t\tsystem status\tnormal 2 28.000000 0 0\trobot status\t326.003968\t39.905332\t11.352600\t-1.618779\t-2.237119\t148.564781\t0.395000\t-0.140000\n\t\n15:30:19.9\tlog_raw\tgps_raw\t#INSPVAXA,USB3,0,47.5,FINESTEERING,2107,282637.900,02008000,471d,15824;INS_ALIGNMENT_COMPLETE,INS_RTKFIXED,37.37049069819,126.72451409261,11.3482,22.3000,0.1872,-0.2201,-0.0214,-1.529619886,-2.288561964,301.270449465,0.4393,0.2929,0.5443,0.1132,0.0922,0.0769,0.0991,0.1040,4.8392,0f000001,0*31e93d15\n\tsystem status\tnormal 2 28.000000 0 0\trobot status\t325.878688\t40.003783\t11.348200\t-1.529620\t-2.288562\t148.729551\t0.274000\t0.037000\n\t\n15:30:20.4\tlog_raw\tgps_raw\t\tsystem status\tnormal 2 28.000000 0 0\trobot status\t325.776588\t40.082900\t11.346000\t-1.463202\t-2.287227\t148.848713\t0.222000\t0.134000\n\t\n15:30:20.9\tlog_raw\tgps_raw\t\tsystem status\tnormal 2 28.000000 0 0\trobot status\t325.665592\t40.168764\t11.343300\t-1.485388\t-2.184363\t149.055795\t0.333000\t-0.029000\n\t\n15:30:21.4\tlog_raw\tgps_raw\t\tsystem status\tnormal 2 27.900000 0 0\trobot status\t325.552763\t40.255679\t11.338200\t-1.377337\t-2.055817\t149.207734\t0.224000\t0.120000\n\t\n15:30:21.9\tlog_raw\tgps_raw\t#INSPVAXA,USB3,0,49.0,FINESTEERING,2107,282639.900,02000000,471d,15824;INS_ALIGNMENT_COMPLETE,INS_RTKFIXED,37.37049383425,126.72450900434,11.3318,22.3000,0.1967,-0.2325,-0.0119,-1.304734991,-1.946875629,300.584763179,0.4389,0.2928,0.5445,0.1134,0.0922,0.0769,0.0991,0.1040,4.8404,0f000001,0*b559a964\n\tsystem status\tnormal 2 27.900000 0 0\trobot status\t325.427977\t40.351855\t11.331800\t-1.304735\t-1.946876\t149.415237\t0.238000\t0.091000\n\t\n15:30:22.4\tlog_raw\tgps_raw\t\tsystem status\tnormal 2 27.900000 0 0\trobot status\t325.326755\t40.429032\t11.327800\t-1.331221\t-1.983649\t149.629824\t0.328000\t-0.037000\n\t\n15:30:22.9\tlog_raw\tgps_raw\t\tsystem status\tnormal 2 27.900000 0 0\trobot status\t325.212739\t40.515603\t11.323300\t-1.367930\t-1.929960\t149.809546\t0.268000\t0.065000\n\t\n15:30:23.4\tlog_raw\tgps_raw\t\tsystem status\tnormal 2 27.900000 0 0\trobot status\t325.098117\t40.603353\t11.319300\t-1.134366\t-1.960291\t149.941691\t0.363000\t-0.101000\n\t\n15:30:23.9\tlog_raw\tgps_raw\t\tsystem status\tnormal 2 27.900000 0 0\trobot status\t324.985443\t40.688483\t11.316200\t-1.094065\t-1.983839\t150.034845\t0.263000\t0.067000\n\t\n15:30:24.4\tlog_raw\tgps_raw\t\tsystem status\tnormal 2 28.000000 0 0\trobot status\t324.870814\t40.771805\t11.311100\t-1.211290\t-2.037909\t150.156431\t0.274000\t0.040000\n\t\n15:30:24.9\tlog_raw\tgps_raw\t#INSPVAXA,USB3,0,51.5,FINESTEERING,2107,282642.900,02000000,471d,15824;INS_ALIGNMENT_COMPLETE,INS_RTKFIXED,37.37049844036,126.72450129803,11.3052,22.3000,0.1790,-0.2238,-0.0065,-1.283994704,-1.940797731,299.771183825,0.4397,0.2927,0.5445,0.1137,0.0922,0.0769,0.0991,0.1039,4.8409,0f000001,0*aafea47d\n\tsystem status\tnormal 2 28.000000 0 0\trobot status\t324.745365\t40.863089\t11.305200\t-1.283995\t-1.940798\t150.228816\t0.351000\t-0.077000\n\t\n15:30:25.4\tlog_raw\tgps_raw\t#INSPVAXA,USB3,0,50.0,FINESTEERING,2107,282643.400,02000000,471d,15824;INS_ALIGNMENT_COMPLETE,INS_RTKFIXED,37.37049919529,126.72450000565,11.2985,22.3000,0.1781,-0.2166,-0.0149,-1.239759750,-1.850856169,299.704406659,0.4403,0.2927,0.5448,0.1137,0.0922,0.0769,0.0991,0.1039,4.8403,0f000001,0*4cea9f21\n\tsystem status\tnormal 2 28.000000 0 0\trobot status\t324.630888\t40.946879\t11.298500\t-1.239760\t-1.850856\t150.295593\t0.265000\t0.052000\n\t\n15:30:25.9\tlog_raw\tgps_raw\t\tsystem status\tnormal 2 28.000000 0 0\trobot status\t324.528397\t41.022844\t11.292100\t-1.110635\t-1.985377\t150.413501\t0.289000\t0.032000\n\t\n15:30:26.4\tlog_raw\tgps_raw\t\tsystem status\tnormal 2 28.000000 0 0\trobot status\t324.412070\t41.105410\t11.286300\t-1.229623\t-2.012181\t150.480057\t0.276000\t0.054000\n\t\n15:30:26.9\tlog_raw\tgps_raw\t#INSPVAXA,USB3,0,50.5,FINESTEERING,2107,282644.900,02000000,471d,15824;INS_ALIGNMENT_COMPLETE,INS_RTKFIXED,37.37050142661,126.72449611592,11.2793,22.3000,0.1856,-0.2171,-0.0219,-1.338634044,-1.925841589,299.522455316,0.4408,0.2928,0.5450,0.1137,0.0922,0.0769,0.0991,0.1039,4.8394,0f000001,0*5553cbbb\n\tsystem status\tnormal 2 28.000000 0 0\trobot status\t324.286342\t41.194534\t11.279300\t-1.338634\t-1.925842\t150.477545\t0.241000\t0.079000\n\t\n15:30:27.4\tlog_raw\tgps_raw\t\tsystem status\tnormal 2 28.000000 0 0\trobot status\t324.182313\t41.270192\t11.275100\t-1.172554\t-1.856540\t150.512182\t0.229000\t0.106000\n\t\n15:30:27.9\tlog_raw\tgps_raw\t\tsystem status\tnormal 2 28.000000 0 0\trobot status\t324.066605\t41.352375\t11.269100\t-1.250534\t-1.720663\t150.539463\t0.225000\t0.111000\n\t\n15:30:28.4\tlog_raw\tgps_raw\t\tsystem status\tnormal 2 28.000000 0 0\trobot status\t323.950455\t41.434814\t11.262800\t-1.275560\t-1.653133\t150.460765\t0.366000\t-0.102000\n\t\n15:30:28.9\tlog_raw\tgps_raw\t\tsystem status\tnormal 2 28.000000 0 0\trobot status\t323.835585\t41.516757\t11.257000\t-1.268227\t-1.520559\t150.427149\t0.255000\t0.062000\n\t\n15:30:29.4\tlog_raw\tgps_raw\t#INSPVAXA,USB3,0,50.5,FINESTEERING,2107,282647.400,02000000,471d,15824;INS_ALIGNMENT_COMPLETE,INS_RTKFIXED,37.37050513933,126.72448960666,11.2512,22.3000,0.1984,-0.2298,-0.0285,-1.166556084,-1.704562940,299.605783810,0.4451,0.2932,0.5473,0.1143,0.0922,0.0771,0.0990,0.1039,4.8365,0f000001,0*2668bb94\n\tsystem status\tnormal 2 28.000000 0 0\trobot status\t323.709762\t41.606611\t11.251200\t-1.166556\t-1.704563\t150.394216\t0.261000\t0.062000\n\t\n15:30:29.9\tlog_raw\tgps_raw\t#INSPVAXA,USB3,0,50.5,FINESTEERING,2107,282647.900,02000000,471d,15824;INS_ALIGNMENT_COMPLETE,INS_RTKFIXED,37.37050588895,126.72448827979,11.2460,22.3000,0.1904,-0.2211,-0.0266,-1.200661987,-1.937489399,299.682292940,0.4451,0.2932,0.5473,0.1143,0.0922,0.0771,0.0990,0.1039,4.8365,0f000001,0*df8b46cf\n\tsystem status\tnormal 2 28.000000 
